vi "Obtain update station config event.vi"(8 "error in":errorcluster) -> (0 "error out":errorcluster, 3 "Update Station config":refnum<user-event>)   [LabVIEW 2018, in "Fiber Auto Collimation References.lvclass"]
doc: "This VI gets the reference to an event that should be fired from the Model loop every time the Station Configuration changes, and sent to the View loops in any running panels to signal a change to any readouts that derive from the Station Configuration."
uses:
  Fiber Auto Collimation References.lvclass
  <userlib>/Recipe/Station Config/Station config.lvclass
  C:/Program Files (x86)/National Instruments/LabVIEW 2018/user.lib/nLight Tidbits/Cross-library references/Cross-library key/Cross-library key.lvclass
  63f3cf25-1f50-4c23-8245-d08426dccd7e.vi
  0414b09b-30d3-4c77-862f-a6629793a3aa.vi
  63f3cf25-1f50-4c23-8245-d08426dccd7e.vi/142acbe8-8303-4e74-9d1e-129091eeaff8.vi
  <userlib>/nLight Tidbits/Cross-library references/Cross-library key/Obtain cross library semaphore and acquire.vi
  63f3cf25-1f50-4c23-8245-d08426dccd7e.vi/bc054919-57c4-4545-b615-452acd1b8a30.vi
  0414b09b-30d3-4c77-862f-a6629793a3aa.vi/62caf744-4864-431d-904f-f381d4d1438f.vi
  0414b09b-30d3-4c77-862f-a6629793a3aa.vi/ed5c71a7-bd36-473c-8e56-3e5fd97c75b2.vi
  <userlib>/nLight Error Handling/Trash error.vi
  <vilib>/Utility/error.llb/Clear Errors.vi
  <vilib>/Utility/semaphor.llb/Obtain Semaphore Reference.vi
  <vilib>/Utility/semaphor.llb/Acquire Semaphore.vi
  <userlib>/nLight Error Handling/Log any errors.vi
  <userlib>/nLight Tidbits/Cross-library references/Cross-library key/Obtain class key.vi
  <vilib>/Utility/semaphor.llb/Release Semaphore.vi
  <vilib>/Utility/semaphor.llb/Release Semaphore Reference.vi
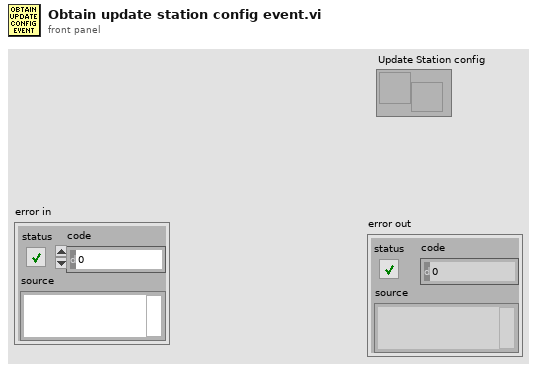
[diagram p1: front panel]
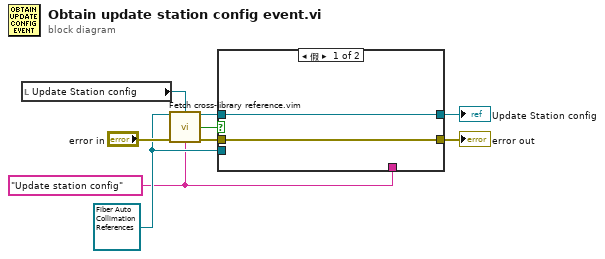
[diagram p0: block diagram]
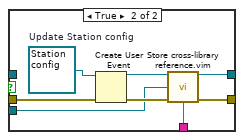
[diagram p2: hidden frame]
diagram:
  w1 = "Update station config"
  w2 = refnum<class "Fiber Auto Collimation References.lvclass"> refnum ("nLight Station Template References.lvclass")
  n1 = local read "Update Station config"() -> (w4:refnum<user-event>)
  n2 = call "Fetch cross-library reference.vim"("Cross-library key"=w2, "Reference type to fetch"=w4, "error in (no error)"="error in", "Specific ref type name [String/Enum]"=w1) -> ("Stored value (if present)"=w3:refnum<user-event>, "Nothing to fetch OR bad reference"=w5:bool, "error out"=w6:errorcluster)  [unwired: 9 in]
  n3 = case shown="假" w5 {
    tunnel: w6 -> [w10 w19]
    tunnel: [w10 w14] -> w8
    tunnel: [w11 w15] -> w9
    tunnel: w3 -> [w11 _]
    tunnel: w2 -> [_ w13]
    tunnel: w1 -> [_ w12]
    frame False {
    }
    frame True {
      w18 = refnum<class "Station config.lvclass"> refnum  # Update Station config
      n4 = Create User Event(user event datatype=w18, error in=w19) -> (user event=w16:refnum<user-event>, error out=w17:errorcluster)
      n5 = call "Store cross-library reference.vim"("Reference to store"=w16, "Cross-library key"=w13, "error in (no error)"=w17, "Specific ref type name [String/Enum]"=w12) -> ("Copy of stored reference"=w15:refnum<user-event>, "error out"=w14:errorcluster)  [unwired: 8 in, 2 out]
    }
  }
  "error out" <- w8
  "Update Station config" <- w9
